vi "json.generate_object.vi"(8 "error in":errorcluster, 11 "ts.epochOfTimeUnit in":refnum<class "ts.epochOfTimeUnit.lvclass">) -> (0 "error out":errorcluster, 2 "JSON Object":string, 3 "ts.epochOfTimeUnit out":refnum<class "ts.epochOfTimeUnit.lvclass">)   [LabVIEW 2018, in "ts.epochOfTimeUnit.lvclass"]
uses:
  ts.epochOfTimeUnit.lvclass
  57b5f462-edfd-4dc3-b983-4b021189c222.vi
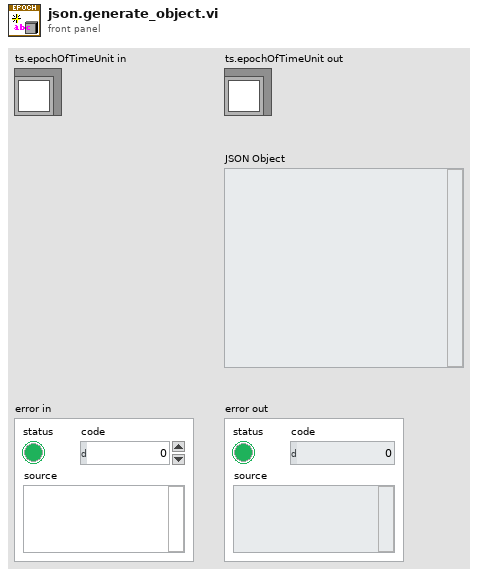
[diagram p1: front panel]
types:
  T1 = cluster{"seriesName":string, "timestampType":cluster{"type":string, "absolute":cluster{"type":string, "epochOfTimeUnit":cluster{"timeUnit":string}}}}
  T2 = enum16{"DAYS", "HOURS", "MINUTES", "SECONDS", "MILLISECONDS", "MICROSECONDS", "NANOSECONDS", "PICOSECONDS"}
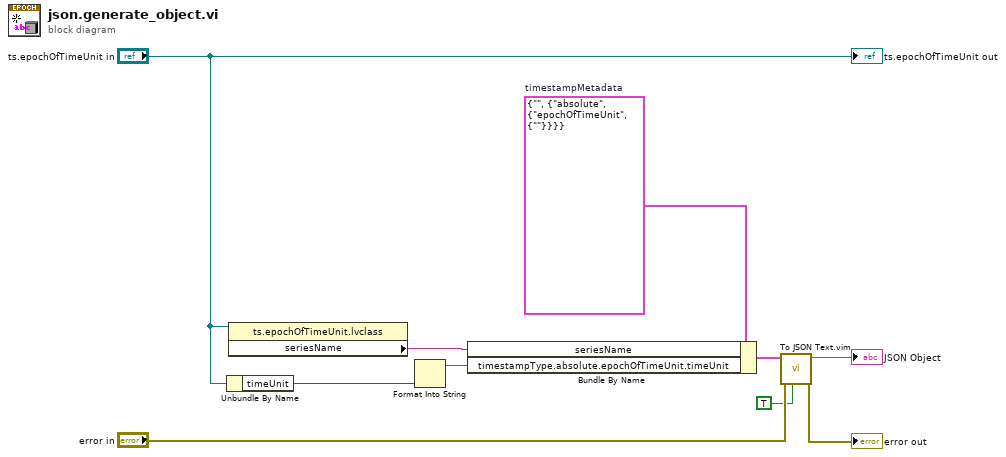
[diagram p0: block diagram]
diagram:
  w1 = T1 {"seriesName"="", "timestampType"={"type"="absolute", "absolute"={"type"="epochOfTimeUnit", "epochOfTimeUnit"={"timeUnit"=""}}}}  # timestampMetadata
  n1 = Unbundle By Name("ts.epochOfTimeUnit in") -> ("timeUnit"=w9:T2)
  n2 = property class="ts.epochOfTimeUnit.lvclass"(reference="ts.epochOfTimeUnit in") -> ("seriesName"=w10:string)  [unwired: 1 in, 2 out]
  n3 = Format Into String(w9) -> (resulting string=w8:string)  [unwired: 3 in, 1 out]
  n4 = Bundle By Name(cluster=w1, "seriesName"=w10, "timestampType.absolute.epochOfTimeUnit.timeUnit"=w8) -> (w7:T1)
  n5 = call "To JSON Text.vim"("Pretty Print?"=TRUE, "error in (no error)"="error in", "Anything"=w7) -> ("error out"=→"error out":errorcluster, "<JSON>"=→"JSON Object":string)  [unwired: 7 in]
  "ts.epochOfTimeUnit out" <- "ts.epochOfTimeUnit in"
